vi "ep_MCSA Spectrum.vi"(0 "signals":dbl[][](array[numeric]), 2 "reset? (F)":bool, 11 "error in (no error)":errorcluster, 12 "initial conditions":T1 {"zoom FFT settings"."FFT settings"."window" items=["Rectangle"=0, "Hanning"=1, "Hamming"=2, "Blackman-Harris"=3, "Exact Blackman"=4, "Blackman"=5, "Flat Top"=6, "4 Term B-Harris "=7, "7 Term B-Harris"=8, "Low Sidelobe"=9, "Blackman Nuttall"=11, "Triangle"=30, "Bartlett-Hanning"=31, "Bohman"=32, "Parzen"=33, "Welch"=34, "Kaiser"=60, "Dolph-Chebyshev"=61, "Gaussian"=62]}) -> (4 "FFT magnitude":cluster{"f0":dbl, "df":dbl, "spectrum":dbl[]}, 6 "FFT phase":cluster{"f0":dbl, "df":dbl, "phase":dbl[]}, 10 "spectrum ready?":bool, 14 "final conditions":T1 {"zoom FFT settings"."FFT settings"."window" items=["Rectangle"=0, "Hanning"=1, "Hamming"=2, "Blackman-Harris"=3, "Exact Blackman"=4, "Blackman"=5, "Flat Top"=6, "4 Term B-Harris "=7, "7 Term B-Harris"=8, "Low Sidelobe"=9, "Blackman Nuttall"=11, "Triangle"=30, "Bartlett-Hanning"=31, "Bohman"=32, "Parzen"=33, "Welch"=34, "Kaiser"=60, "Dolph-Chebyshev"=61, "Gaussian"=62]}, 15 "error out":errorcluster)   [LabVIEW 2014, in "NI_EP_Motor Monitoring.lvlib"]
uses:
  <vilib>/addons/Electrical Power/Motor Monitoring/NI_EP_Motor Monitoring.lvlib
  <vilib>/addons/Electrical Power/Motor Monitoring/subVIs/ep_Initial Conditions for MCSA Spectra.ctl
  <vilib>/addons/Electrical Power/Motor Monitoring/subVIs/ep_Demodulation Algorithm.ctl
  <vilib>/addons/Electrical Power/Motor Monitoring/subVIs/ep_Zoom FFT Settings.ctl
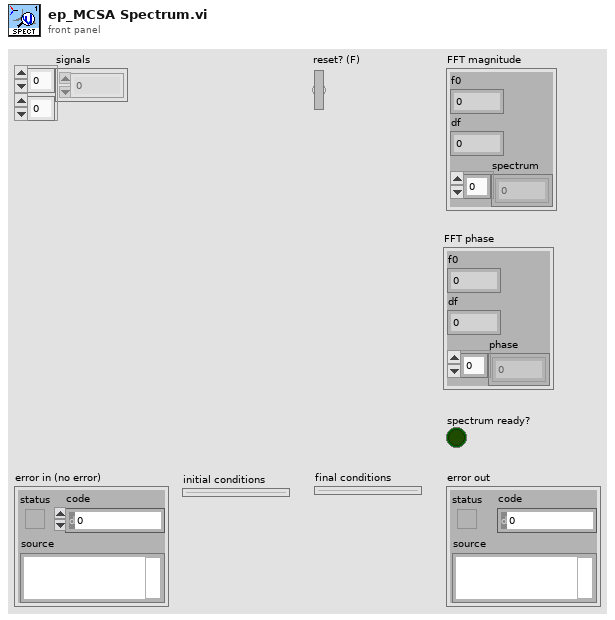
[diagram p1: front panel]
types:
  T1 = typedef "NI_EP_Motor Monitoring.lvlib/ep_Initial Conditions for MCSA Spectra.ctl" = cluster{"hilbert state":cluster{"delay conditions":dbl[], "filter conditions":dbl[]}, "zoom FFT state":cluster{"phase state":dbl, "zoom FFT state":cluster{"zoom settings state":cluster{"zoom":i32, "stop band attenuation":enum16{"84 dB", "96 dB", "120 dB"}, "alias protect in final transition":bool, "oversampling ratio":dbl}, "SML Decimation Filter (complex input) state":cluster{"decimation settings state":cluster{"M":i32, "stop band attenuation":enum16{"84 dB", "96 dB", "120 dB"}, "alias protect in transition band":bool, "oversampling ratio":dbl}, "counter for garbage samples state":i32, "sml_Parameter Setting for Zoom Factor state":cluster{"filter length * interpolation state":i32, "interpolation state":i32, "comb filter order state":i32, "CFIR par state":cluster{"h":dbl[], "M":i32, "N":i32}, "LFIR par state":cluster{"h":dbl[], "M":i32, "N":i32}, "CIC Stages state":i32}, "aal_CIC (complex input) state":cluster{"aal_cascaded moving average (complex input) state":cluster{"states":cdb[], "circular buffers state":cdb[][], "circular buffer counter state":i32}, "aal_moving average with decimation by order (complex input) state":cluster{"residue result state":cdb, "processed data counter state":i32}}, "sml_Cascaded Decimation Filter (complex input) CFIR state":cluster{"unprocessed data state":cdb[], "final conditions state":cdb[][], "sml_M-1 Decimator with IC (complex input) state":cluster{"coefficients in reverse order state":dbl[], "max index for coefficients state":i32}}, "sml_Cascaded Decimation Filter (complex input) LFIR state":cluster{"unprocessed data state":cdb[], "final conditions state":cdb[][], "sml_M-1 Decimator with IC (complex input) state":cluster{"coefficients in reverse order state":dbl[], "max index for coefficients state":i32}}}, "ma_SML Data Packing (complex input) state":cluster{"array getting packed state":cdb[], "last array processed state":cdb[], "index state":i32, "packing parameters state":cluster{i32, "size":i32}}}, "FFT{X} [Vrms]":cdb[]}, "IIR filter state":cluster{"filter state":dbl[]}, "demodulation settings":cluster{"enable? (F)":bool, "algorithm":T2}, "highpass IIR Filter":cluster{"filter structure":enum32{"IIR 2nd Order", "IIR 4th Order"}, "Reverse Coefficients":dbl[], "Forward Coefficients":dbl[]}, "Hilbert FIR filter":cluster{"coefficients":dbl[], "delay":i32}, "zoom FFT settings":T3}
  T2 = typedef "NI_EP_Motor Monitoring.lvlib/ep_Demodulation Algorithm.ctl" = enum16{"1-phase signal", "3-phase signals"}
  T3 = typedef "NI_EP_Motor Monitoring.lvlib/ep_Zoom FFT Settings.ctl" = cluster{"FFT settings":cluster{"window":u16, "Window Size":i32, "FFT Size":i32, "%overlap":dbl}, "zoom settings":cluster{"zoom":i32, "stop band attenuation":enum16{"84 dB", "96 dB", "120 dB"}, "alias protect in final transition":bool, "oversampling ratio":dbl}, "other settings":cluster{"fmod":dbl, "f0":dbl, "df":dbl, "oidx":i32, "olen":i32}, "iterations":i32, "max block size":i32, "fs":dbl}
  T4 = cluster{"filter structure":enum32{"IIR 2nd Order", "IIR 4th Order"}, "Reverse Coefficients":dbl[], "Forward Coefficients":dbl[]}
  T5 = cluster{"delay conditions":dbl[], "filter conditions":dbl[]}
  T6 = cluster{"phase state":dbl, "zoom FFT state":cluster{"zoom settings state":cluster{"zoom":i32, "stop band attenuation":enum16{"84 dB", "96 dB", "120 dB"}, "alias protect in final transition":bool, "oversampling ratio":dbl}, "SML Decimation Filter (complex input) state":cluster{"decimation settings state":cluster{"M":i32, "stop band attenuation":enum16{"84 dB", "96 dB", "120 dB"}, "alias protect in transition band":bool, "oversampling ratio":dbl}, "counter for garbage samples state":i32, "sml_Parameter Setting for Zoom Factor state":cluster{"filter length * interpolation state":i32, "interpolation state":i32, "comb filter order state":i32, "CFIR par state":cluster{"h":dbl[], "M":i32, "N":i32}, "LFIR par state":cluster{"h":dbl[], "M":i32, "N":i32}, "CIC Stages state":i32}, "aal_CIC (complex input) state":cluster{"aal_cascaded moving average (complex input) state":cluster{"states":cdb[], "circular buffers state":cdb[][], "circular buffer counter state":i32}, "aal_moving average with decimation by order (complex input) state":cluster{"residue result state":cdb, "processed data counter state":i32}}, "sml_Cascaded Decimation Filter (complex input) CFIR state":cluster{"unprocessed data state":cdb[], "final conditions state":cdb[][], "sml_M-1 Decimator with IC (complex input) state":cluster{"coefficients in reverse order state":dbl[], "max index for coefficients state":i32}}, "sml_Cascaded Decimation Filter (complex input) LFIR state":cluster{"unprocessed data state":cdb[], "final conditions state":cdb[][], "sml_M-1 Decimator with IC (complex input) state":cluster{"coefficients in reverse order state":dbl[], "max index for coefficients state":i32}}}, "ma_SML Data Packing (complex input) state":cluster{"array getting packed state":cdb[], "last array processed state":cdb[], "index state":i32, "packing parameters state":cluster{i32, "size":i32}}}, "FFT{X} [Vrms]":cdb[]}
  T7 = cluster{"filter conditions":dbl[], "delay conditions":dbl[]}
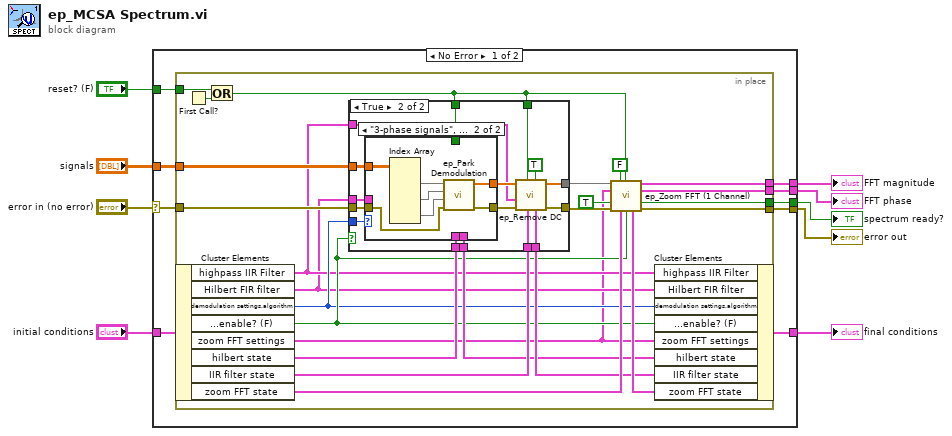
[diagram p0: block diagram]
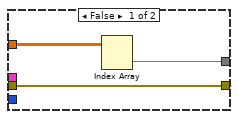
[diagram p2: hidden frame]
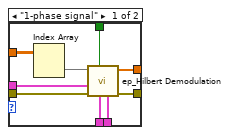
[diagram p3: hidden frame]
diagram:
  n1 = case shown="No Error" "error in (no error)" {
    selector: "error in (no error)" -> [w18 w78]
    tunnel: [w17 w78] -> w8
    tunnel: [w13 _] -> w7
    tunnel: [w14 _] -> w6
    tunnel: [w10 _] -> w2
    tunnel: "initial conditions" -> [w11 _]
    tunnel: "signals" -> [w16 _]
    tunnel: "reset? (F)" -> [w15 _]
    tunnel: [w12 _] -> w1
    frame No Error {
      n2 = in-place {
        in-place-border: w18 -> [w39]
        in-place-border: [w38] -> w17
        in-place-border: w16 -> [w37]
        in-place-border: w15 -> [w35]
        in-place-border: [w34] -> w14
        in-place-border: [w32] -> w13
        in-place-border: [w31] -> w12
        n3 = in-place-cluster #1(w11) -> ("highpass IIR Filter"=w21:T4, "Hilbert FIR filter"=w20:cluster{"coefficients":dbl[], "delay":i32}, "demodulation settings.algorithm"=w22:T2, "demodulation settings.enable? (F)"=w23:bool, "zoom FFT settings"=w19:T3, "hilbert state"=w25:T5, "IIR filter state"=w27:cluster{"filter state":dbl[]}, "zoom FFT state"=w29:T6)
        n4 = First Call?() -> (First Call?: T/F=w36:bool)
        n5 = Or(x=w35, y=w36) -> (x .or. y?=w33:bool)
        n6 = case shown="True" w23 {
          tunnel: w37 -> [w45 w61]
          tunnel: w39 -> [w43 w60]
          tunnel: [w44 w58] -> w40
          tunnel: [w43 w48] -> w42
          tunnel: w22 -> [_ w59]
          tunnel: w20 -> [_ w57]
          tunnel: w33 -> [_ w56]
          tunnel: w25 -> [_ w55]
          tunnel: [_ w54] -> w24
          tunnel: w33 -> [_ w47]
          tunnel: w27 -> [_ w53]
          tunnel: [_ w52] -> w26
          tunnel: w21 -> [_ w50]
          frame False {
            n7 = Index Array(array=w45) -> (element=w44:dbl[])  [unwired: 2 in]
          }
          frame True {
            n8 = case shown="\"3-phase signals\", Default" w59 {
              tunnel: w61 -> [w70 w77]
              tunnel: [w66 w72] -> w51
              tunnel: w60 -> [w68 w73]
              tunnel: [w67 w71] -> w49
              tunnel: w57 -> [w65 _]
              tunnel: w56 -> [w64 _]
              tunnel: w55 -> [w63 _]
              tunnel: [w62 _] -> w54
              frame "1-phase signal" {
                n9 = Index Array(array=w70) -> (element=w69:dbl[])  [unwired: 2 in]
                n10 = call <vilib>:"ep_Hilbert Demodulation.vi"("previous state"=w63, "reset? (F)"=w64, "error in (no error)"=w68, "filter information"=w65, "signal"=w69) -> ("error out"=w67:errorcluster, "demodulated signal"=w66:dbl[], "next state"=w62:T7)  [unwired: 4 in]
              }
              frame "3-phase signals", Default {
                n11 = Index Array(array=w77) -> (element #1=w76:dbl[], element #2=w74:dbl[], element #3=w75:dbl[])  [unwired: 6 in]
                n12 = call <vilib>:"ep_Park Demodulation.vi"("error in (no error)"=w73, "phase C"=w75, "phase B"=w74, "phase A"=w76) -> ("error out"=w71:errorcluster, "demodulated signal"=w72:dbl[])  [unwired: 6 in]
              }
            }
            n13 = call <vilib>:"ep_Remove DC.vi"("enable? (T)"=TRUE, "IIR filter state in"=w53, "reset? (F)"=w47, "error in (no error)"=w49, "highpass IIR filter"=w50, "signal in"=w51) -> ("error out"=w48:errorcluster, "signal out"=w58:dbl[], "IIR filter state out"=w52:cluster{"filter state":dbl[]})  [unwired: 3 in]
          }
        }
        n14 = call <vilib>:"ep_Zoom FFT (1 Channel).vi"("signal"=w40, "phase output? (F)"=FALSE, "reset? (F)"=w33, "zoom FFT settings"=w19, "dB on? (T)"=TRUE, "error in (no error)"=w42, "zoom FFT state in"=w29, "demodulated? (F)"=w23) -> ("FFT magnitude"=w34:cluster{"f0":dbl, "df":dbl, "magnitude":dbl[]}, "FFT phase"=w31:cluster{"f0":dbl, "df":dbl, "phase":dbl[]}, "spectrum ready?"=w32:bool, "zoom FFT state out"=w28:T6, "error out"=w38:errorcluster)  [unwired: 3 in]
        n15 = in-place-cluster #1("highpass IIR Filter"=w21, "Hilbert FIR filter"=w20, "demodulation settings.algorithm"=w22, "demodulation settings.enable? (F)"=w23, "zoom FFT settings"=w19, "hilbert state"=w24, "IIR filter state"=w26, "zoom FFT state"=w28) -> (w10:T1)
      }
    }
    frame Error {
    }
  }
  "error out" <- w8
  "spectrum ready?" <- w7
  "FFT magnitude" <- w6
  "final conditions" <- w2
  "FFT phase" <- w1
